vi "Sour_Meas_Instrument.vi"(0 "Command":string="SOURce:VOLTage:DC 10", 11 "Error_In":errorcluster) -> (4 "Responce":dbl, 6 "Action":string, 8 "Parameter":string, 15 "Error_Out":errorcluster)   [LabVIEW 2021]
doc: "This VI SOURce and MEASure the data with the command provided.\nSOURce- Storing the data into the INI file.\nMEASure - Retrieving the data from the INI file."
uses:
  <vilib>/Utility/config.llb/NI_LVConfig.lvlib
  <vilib>/Utility/config.llb/Read Key (Double).vi
  <vilib>/Utility/config.llb/Write Key (Double).vi
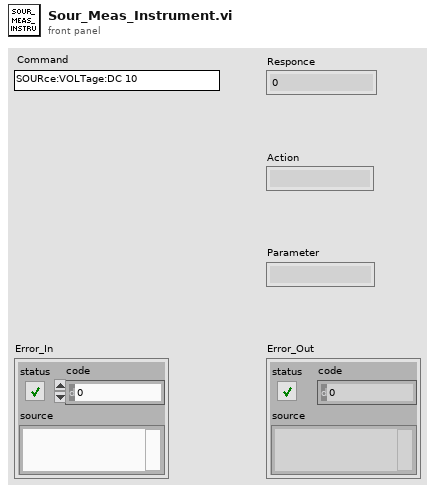
[diagram p1: front panel]
types:
  T1 = typedef "NI_LVConfig.lvlib/Config Data RefNum.ctl" = refnum<k1>
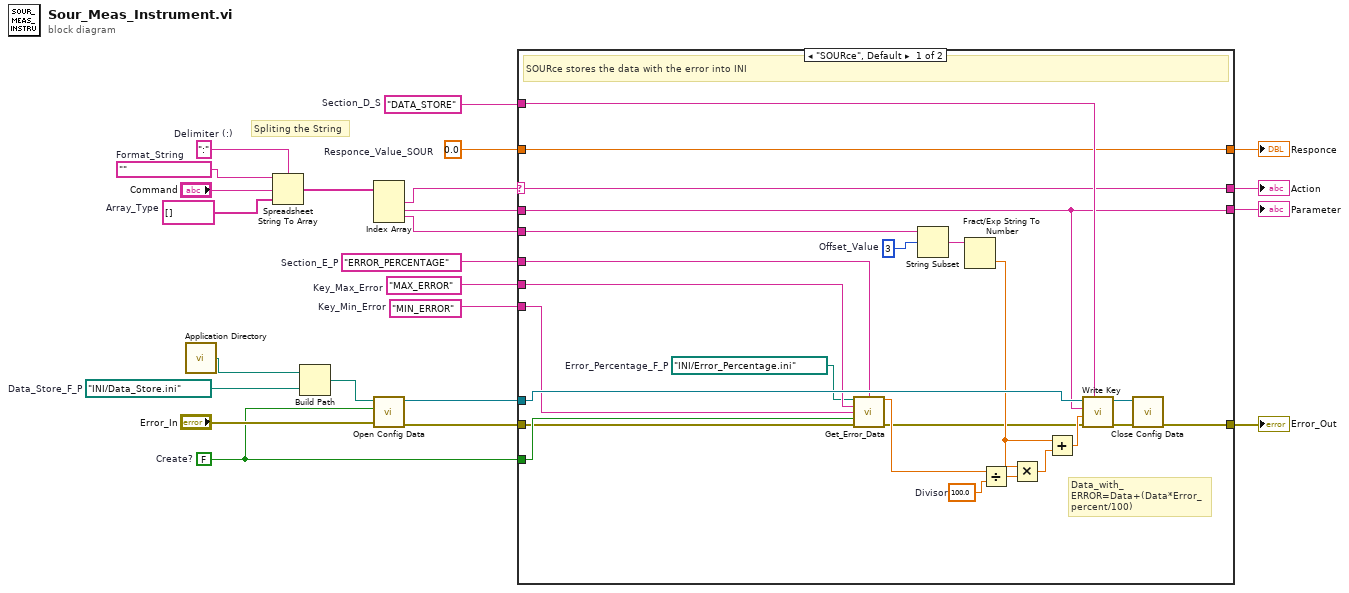
[diagram p0: block diagram]
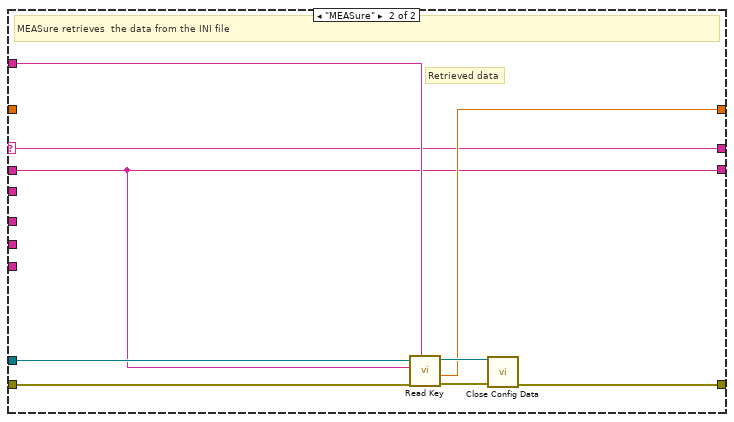
[diagram p2: hidden frame]
diagram:
  w7 = 0.0  # Responce_Value_SOUR
  w11 = "MIN_ERROR"  # Key_Min_Error
  w12 = "MAX_ERROR"  # Key_Max_Error
  w13 = "ERROR_PERCENTAGE"  # Section_E_P
  w4 = FALSE  # Create?
  w14 = "DATA_STORE"  # Section_D_S
  w1 = path "INI/Data_Store.ini"  # Data_Store_F_P
  w21 = ""  # Format_String
  w24 = string[] []  # Array_Type
  w22 = ":"  # Delimiter (:)
  # "Spliting the String"
  n1 = call <vilib>:"Application Directory.vi"() -> ("Application Directory"=w2:path)
  n2 = Spreadsheet String To Array(delimiter (Tab)=w22, format string=w21, spreadsheet string="Command", array type (2D Dbl)=w24) -> (array=w19:string[])
  n3 = Build Path(base path=w2, name or relative path=w1) -> (appended path=w3:path)
  n4 = Index Array(array=w19) -> (element #1=w20:string, element #2=w18:string, element #3=w17:string)  [unwired: 3 in]
  n5 = call <vilib>:"Open Config Data.vi"("error in (no error)"="Error_In", "create file if necessary (T)"=w4, "configuration file path"=w3) -> ("error out"=w16:errorcluster, "refnum"=w15:T1)  [unwired: 6 in, 1 out]
  n6 = case shown="\"SOURce\", Default" w20 {
    selector: w20 -> [w35 w51]
    tunnel: w18 -> [w34 w50]
    tunnel: w17 -> [w30 _]
    tunnel: w16 -> [w27 w55]
    tunnel: w15 -> [w48 w56]
    tunnel: w14 -> [w41 w57]
    tunnel: [w33 w52] -> w6
    tunnel: w13 -> [w40 _]
    tunnel: w12 -> [w38 _]
    tunnel: w11 -> [w39 _]
    tunnel: [w25 w49] -> w10
    tunnel: [w35 w51] -> w9
    tunnel: [w34 w50] -> w8
    tunnel: w7 -> [w33 _]
    tunnel: w4 -> [w29 _]
    frame "SOURce", Default {
      w28 = path "INI/Error_Percentage.ini"  # Error_Percentage_F_P
      w36 = 100.0  # Divisor
      w31 = 3  # Offset_Value
      # "Data_with_ERROR=Data+(Data*Error_percent/100)"
      # "SOURce stores the data with the error into INI"
      n7 = call "Get_Error_Data.vi"("Error_Percentage_F_P"=w28, "Section_E_P"=w40, "Key_Max_Error"=w38, "Key_Min_Error"=w39, "Create?"=w29, "Error_In"=w27) -> ("Error_Data"=w37:dbl, "Error_Out"=w26:errorcluster)  [unwired: 8 in]
      n8 = String Subset(string=w30, offset (0)=w31) -> (substring=w32:string)  [unwired: 1 in]
      n9 = Fract/Exp String To Number(string=w32) -> (number=w45:dbl)  [unwired: 3 in, 1 out]
      n10 = Divide(x=w37, y=w36) -> (x/y=w47:dbl)
      n11 = Multiply(x=w45, y=w47) -> (x*y=w46:dbl)
      n12 = Add(x=w45, y=w46) -> (x+y=w44:dbl)
      n13 = call-poly <vilib>:"Write Key.vi"("section"=w41, "error in (no error)"=w26, "value"=w44, "key"=w34, "refnum"=w48) -> ("error out"=w42:errorcluster, "refnum out"=w43:T1)  [unwired: 4 in, 1 out]
      n14 = call <vilib>:"Close Config Data.vi"("error in (no error)"=w42, "refnum"=w43) -> ("error out"=w25:errorcluster)  [unwired: 8 in, 1 out]
    }
    frame "MEASure" {
      # "Retrieved data"
      # "MEASure retrieves  the data from the INI file"
      n15 = call-poly <vilib>:"Read Key.vi"("section"=w57, "error in (no error)"=w55, "key"=w50, "refnum"=w56) -> ("error out"=w53:errorcluster, "value"=w52:dbl, "refnum out"=w54:T1)  [unwired: 4 in, 1 out]
      n16 = call <vilib>:"Close Config Data.vi"("error in (no error)"=w53, "refnum"=w54) -> ("error out"=w49:errorcluster)  [unwired: 8 in, 1 out]
    }
  }
  "Responce" <- w6
  "Error_Out" <- w10
  "Action" <- w9
  "Parameter" <- w8
